vi "statsCalcWithSubVI.vi"() -> ()   [LabVIEW 2014]
uses:
  <vilib>/gmath/statdist.llb/Normal Random.vi
  <userlib>/StatsCalculatorLabView/StatsCalculatorLabView.lvlib
  <vilib>/gmath/NI_Gmath.lvlib
  <vilib>/Analysis/NI_AALBase.lvlib
panel:
  in  "Output\nFilename":string="statsSummary.txt"
  out "Gaussian Distribution":T1(graph)
  out "Error State":errorcluster
  out "Standard Deviation":dbl(knob) scale=0.0..10.0
  out "Mean":dbl(knob) scale=0.0..10.0
  out "Sum":dbl(knob) scale=0.0..10.0
  in  "True\nStandard Deviation":dbl(knob)=0.5 scale=0.5..2.0
  in  "True Mean":dbl(knob) scale=-5.0..5.0
  in  "Number of Values":i32(knob)=50 scale=100.0..1000.0
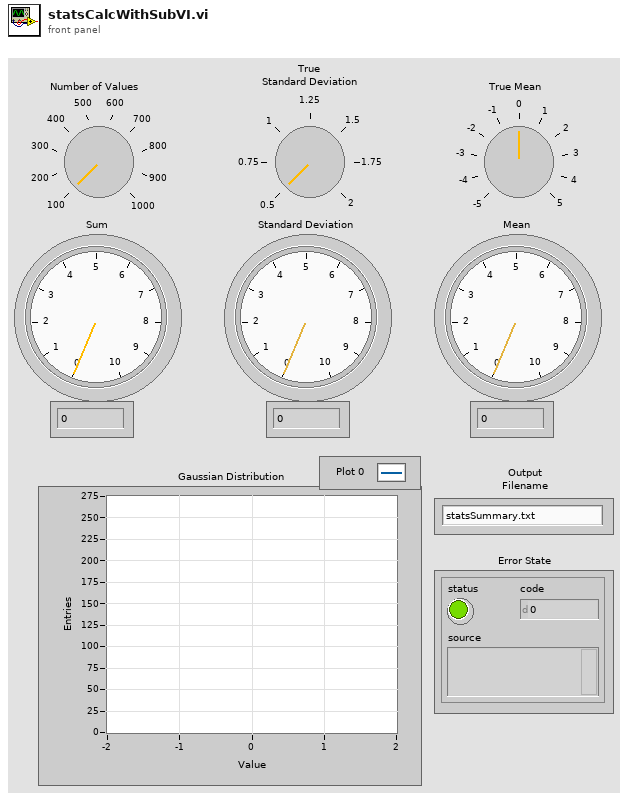
[diagram p1: front panel]
types:
  T1 = cluster{"X Values":dbl[], "Histogram: h(x)":i32[]}
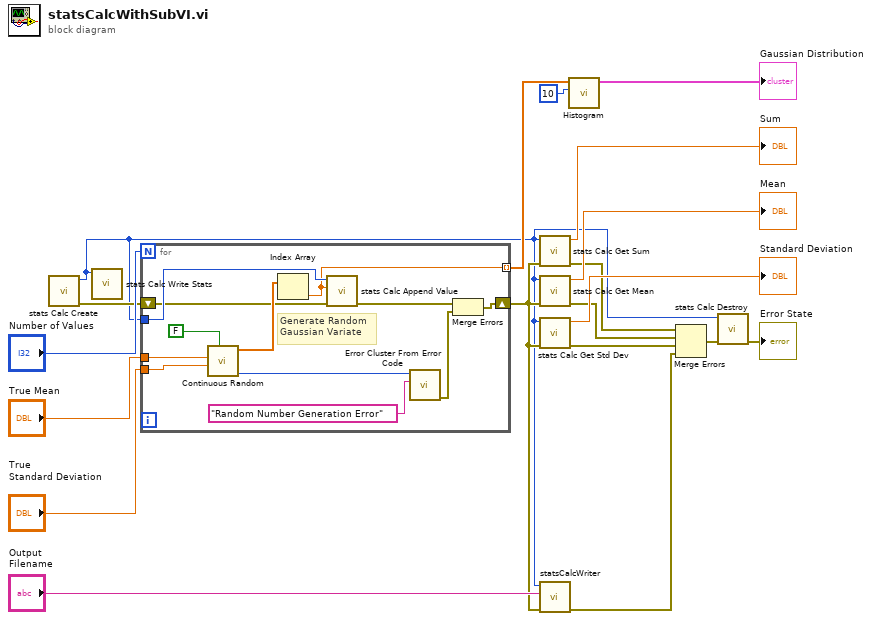
[diagram p0: block diagram]
diagram:
  n1 = call <userlib>:"stats Calc Create.vi"() -> ("error out"=w16:errorcluster, "function return"=w2:i32)  [unwired: 10 in]
  n2 = call <userlib>:"stats Calc Write Stats.vi"("handle"=w2) -> ()  [unwired: 10 in, 1 out]
  n3 = for {
    N: "Number of Values" -> [_]
    tunnel: w2 -> [w31]
    tunnel: "True\nStandard Deviation" -> [w30]
    tunnel: "True Mean" -> [w29]
    shift-right: [w21] -> w3
    shift-left: w16 -> [w24]
    tunnel: [w20] -> w7 mode=indexing
    # "Generate Random\nGaussian Variate"
    n4 = call-poly <vilib>:"Continuous Random.vi"("reset"=FALSE, "std"=w30, "mean"=w29) -> ("error"=w26:i32, "normal random data"=w27:dbl[])  [unwired: 7 in]
    n5 = Index Array(array=w27) -> (element=w20:dbl)  [unwired: 1 in]
    n6 = call <userlib>:"stats Calc Append Value.vi"("error in (no error)"=w24, "value"=w20, "handle"=w31) -> ("error out"=w22:errorcluster)  [unwired: 8 in]
    n7 = call <vilib>:"Error Cluster From Error Code.vi"("error message (\"\")"="Random Number Generation Error", "error code (0)"=w26) -> ("error out"=w23:errorcluster)  [unwired: 7 in]
    n8 = Merge Errors(w22, w23) -> (w21:errorcluster)
  }
  n9 = call <userlib>:"stats Calc Get Sum.vi"("error in (no error)"=w3, "handle"=w2) -> ("error out"=w12:errorcluster, "function return"=→"Sum":dbl)  [unwired: 8 in]
  n10 = call <userlib>:"stats Calc Get Mean.vi"("error in (no error)"=w3, "handle"=w2) -> ("error out"=w11:errorcluster, "function return"=→"Mean":dbl)  [unwired: 8 in]
  n11 = call <userlib>:"stats Calc Get Std Dev.vi"("error in (no error)"=w3, "handle"=w2) -> ("error out"=w10:errorcluster, "function return"=→"Standard Deviation":dbl)  [unwired: 8 in]
  n12 = call "statsCalcWriter.vi"("error in (no error)"=w3, "Output\nFilename"="Output\nFilename", "StatsCalc ID"=w2) -> ("error out"=w1:errorcluster)  [unwired: 8 in]
  n13 = call <vilib>:"Histogram.vi"("intervals"=10, "X"=w7) -> ("Histogram Graph"=→"Gaussian Distribution":T1)  [unwired: 6 in, 3 out]
  n14 = Merge Errors(w12, w11, w10, w1) -> (w9:errorcluster)
  n15 = call <userlib>:"stats Calc Destroy.vi"("error in (no error)"=w9, "handle"=w2) -> ("error out"=→"Error State":errorcluster)  [unwired: 9 in]
